vi "Sea-Level SWI Get Adapter State.vi"(8 "error in (no error)":errorcluster, 11 "Handle":i32) -> (0 "error out":errorcluster, 2 "Adapter State":T1, 3 "Handle Out":i32, 4 "Error Code":T2=enum."SEAIO_ERROR_BUSY")   [LabVIEW 2011]
uses:
  TypeDefs/Sea-Level SWI Error Code.ctl
  TypeDefs/Sea-Level SWI Adapter State.ctl
  SeaIo32.dll
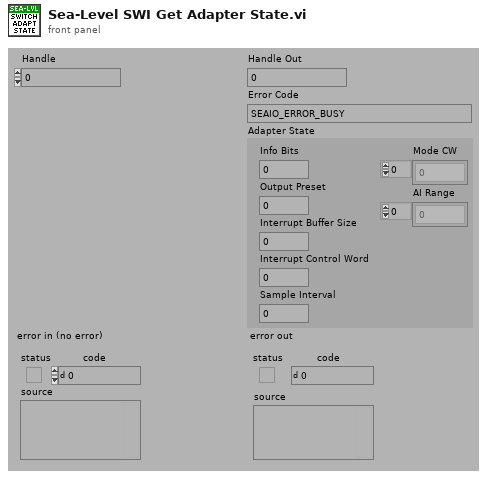
[diagram p1: front panel]
types:
  T1 = typedef "Sea-Level SWI Adapter State.ctl" = cluster{"Info Bits":i32, "Output Preset":i32, "Interrupt Buffer Size":i32, "Interrupt Control Word":i32, "Sample Interval":i32, "Mode CW":i8[], "AI Range":i8[]}
  T2 = typedef "Sea-Level SWI Error Code.ctl" = enum16{"SEAIO_ERROR_NONE", "SEAIO_ERROR_PARAM", "SEAIO_ERROR_NOT_SUPPORTED", "SEAIO_ERROR_PORT_NOT_OPEN", "SEAIO_ERROR_INVALID_NAME", "SEAIO_ERROR_SHARING_VIOLATION", "SEAIO_ERROR_DRIVER_TYPE", "SEAIO_ERROR_BUFFER", "SEAIO_ERROR_INCOMPLETE", "SEAIO_ERROR_GENERAL", "SEAIO_ERROR_IO_PENDING", "SEAIO_ERROR_NO_TXBUFFER", "SEAIO_ERROR_INVALID_DEVICE_REQUEST", "SEAIO_ERROR_INVALID_HANDLE", "SEAIO_ERROR_CANCELED", "SEAIO_ERROR_LAST", "SEAIO_ERROR_NO_MEMORY", "SEAIO_ERROR_BUSY"}
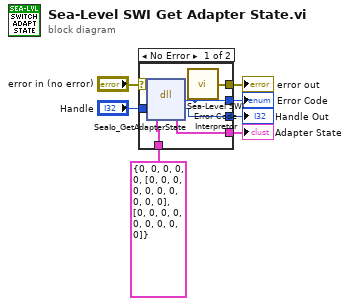
[diagram p0: block diagram]
diagram:
  n1 = case shown="No Error" "error in (no error)" {
    selector: "error in (no error)" -> [_ w15]
    tunnel: [w13 _] -> w7
    tunnel: [w12 w15] -> w6
    tunnel: "Handle" -> [w11 w14]
    tunnel: [w9 w14] -> w2
    tunnel: T1 {"Info Bits"=0, "Output Preset"=0, "Interrupt Buffer Size"=0, "Interrupt Control Word"=0, "Sample Interval"=0, "Mode CW"=[0, 0, 0, 0, 0, 0, 0, 0, 0, 0], "AI Range"=[0, 0, 0, 0, 0, 0, 0, 0, 0]} ("Adapter State") -> [w10 _]
    tunnel: [w8 _] -> w1
    frame No Error {
      n2 = dll-call lib="C:/Development/Spartan/www/drivers/SWI/Sea-Level/SeaIo32.dll" fn="SeaIo_GetAdapterState"("Handle"=w11, "Adapter State"=w10) -> ("Error Code"=w13:i32, "Handle"=w9:i32, "Adapter State"=w8:T1)  [unwired: 3 in, 2 out]
      n3 = call "Sea-Level SWI Error Code Interpretor.vi"("Error Code"=w13) -> ("error out"=w12:errorcluster)
    }
    frame Error {
    }
  }
  "Error Code" <- w7
  "error out" <- w6
  "Adapter State" <- w1
  "Handle Out" <- w2
